vi "Connect.vi"(0 "Credentials":T1, 1 "Authenticate":bool=TRUE, 3 "error in (no error)":errorcluster) -> (6 "connection ID out":refnum<k5>, 7 "Connection Status":T4=enum."Connection refused: not authorized", 9 "error out":errorcluster)   [LabVIEW 2013, in "IOTFoundation.lvlib"]
uses:
  IOTFoundation.lvlib
  Controls/Connection_Return_Codes.ctl
  Controls/MessageType.ctl
  Controls/QoS.ctl
panel:
  out "QoS Level":T2
  out "MessageType":T3
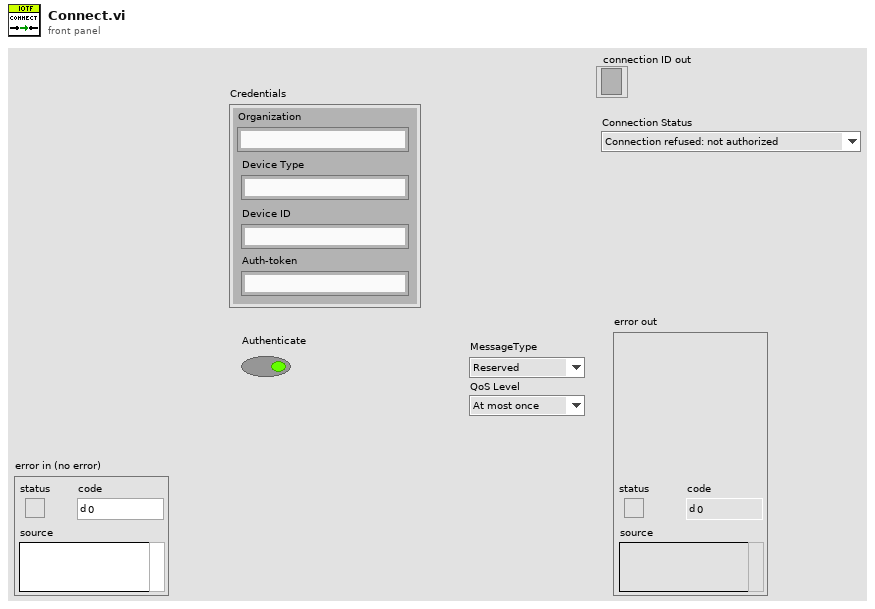
[diagram p1: front panel]
types:
  T1 = cluster{"Organization":string, "Device Type":string, "Device ID":string, "Auth-token":string}
  T2 = typedef "IOTFoundation.lvlib/QoS.ctl" = enum8{"At most once", "At least once", "Exactly once", "Reserved"}
  T3 = typedef "IOTFoundation.lvlib/MessageType.ctl" = enum32{"Reserved", "CONNECT", "CONNACK", "PUBLISH", "PUBACK", "PUBREC", "PUBREL", "PUBCOMP", "SUBSCRIBE", "SUBACK", "UNSUBSCRIBE", "UNSUBACK", "PINGREQ", "PINGRESP", "DISCONNECT", "Reserved2"}
  T4 = typedef "IOTFoundation.lvlib/Connection_Return_Codes.ctl" = enum16{"Connection accepted", "Connection refused: unacceptable protocol version", "Connection refused: identifier rejected", "Connection refused: Server unavailable", "Connection refused: bad user name or password", "Connection refused: not authorized"}
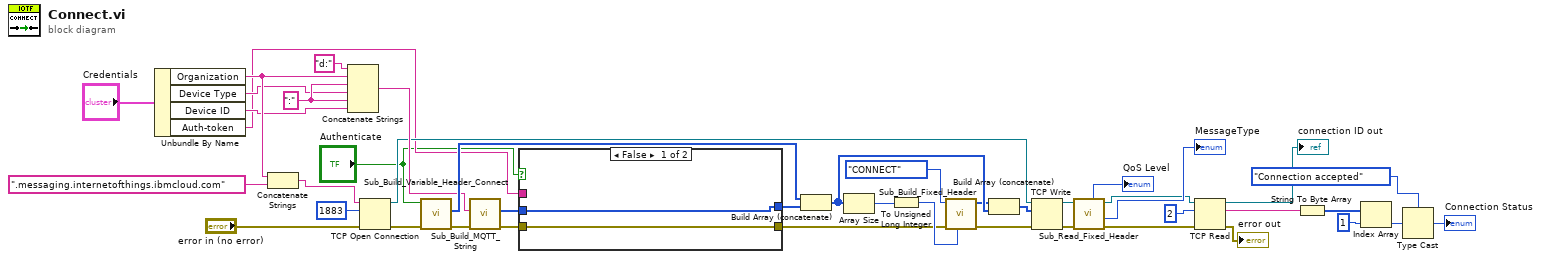
[diagram p0: block diagram]
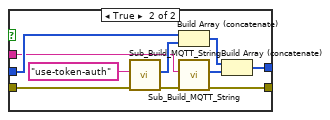
[diagram p2: hidden frame]
diagram:
  w30 = ":"
  n1 = Unbundle By Name("Credentials") -> ("Organization"=w5:string, "Device Type"=w4:string, "Device ID"=w3:string, "Auth-token"=w2:string)
  n2 = Concatenate Strings(w5, ".messaging.internetofthings.ibmcloud.com") -> (w26:string)
  n3 = Concatenate Strings("d:", w5, w30, w4, w30, w3) -> (w29:string)
  n4 = TCP Open Connection(address=w26, remote port or service name=1883, error in (no error)="error in (no error)") -> (connection ID=w23:refnum<k5>, error out=w27:errorcluster)  [unwired: 2 in]
  n5 = call "Sub_Build_Variable_Header_Connect.vi"("error in (no error)"=w27, "Authenticate"="Authenticate") -> ("error out"=w42:errorcluster, "Variable Header"=w41:u8[])  [unwired: 8 in]
  n6 = call "Sub_Build_MQTT_String.vi"("error in (no error)"=w42, "String to be encoded"=w29) -> ("error out"=w35:errorcluster, "UTF8 Byte Array"=w36:u8[])  [unwired: 8 in]
  n7 = case shown="False" "Authenticate" {
    tunnel: w36 -> [w44 w54]
    tunnel: w35 -> [w45 w53]
    tunnel: [w44 w49] -> w34
    tunnel: [w45 w48] -> w33
    tunnel: w2 -> [_ w47]
    frame False {
    }
    frame True {
      n8 = call "Sub_Build_MQTT_String.vi"("error in (no error)"=w53, "String to be encoded"="use-token-auth") -> ("error out"=w52:errorcluster, "UTF8 Byte Array"=w55:u8[])  [unwired: 8 in]
      n9 = Build Array (concatenate)(w54, w55) -> (w51:u8[])
      n10 = call "Sub_Build_MQTT_String.vi"("error in (no error)"=w52, "String to be encoded"=w47) -> ("error out"=w48:errorcluster, "UTF8 Byte Array"=w50:u8[])  [unwired: 8 in]
      n11 = Build Array (concatenate)(w51, w50) -> (w49:u8[])
    }
  }
  n12 = Build Array (concatenate)(w41, w34) -> (w40:u8[])
  n13 = Array Size(array=w40) -> (size(s)=w38:i32)
  n14 = To Unsigned Long Integer(number=w38) -> (unsigned 32bit integer=w37:u32)
  n15 = call "Sub_Build_Fixed_Header.vi"("Remaining Length"=w37, "error in (no error)"=w33, "MessageType"=MessageType."CONNECT") -> ("error out"=w24:errorcluster, "Fixed Header"=w39:u8[])  [unwired: 7 in]
  n16 = Build Array (concatenate)(w39, w40) -> (w22:u8[])
  n17 = TCP Write(connection ID=w23, data in=w22, error in (no error)=w24) -> (connection ID out=w11:refnum<k5>, error out=w10:errorcluster)  [unwired: 1 in, 1 out]
  n18 = call "Sub_Read_Fixed_Header.vi"("error in (no error)"=w10, "connection ID"=w11) -> ("error out"=w14:errorcluster, "MessageType"=→"MessageType":T3, "connection ID out"=w13:refnum<k5>, "QoS Level"=→"QoS Level":T2)  [unwired: 3 in, 3 out]
  n19 = TCP Read(connection ID=w13, bytes to read=2, error in (no error)=w14) -> (connection ID out=→"connection ID out":refnum<k5>, data out=w12:string, error out=→"error out":errorcluster)  [unwired: 2 in]
  n20 = String To Byte Array(string=w12) -> (unsigned byte array=w16:u8[])
  n21 = Index Array(array=w16, index=1) -> (element=w21:u8)
  n22 = Type Cast(type=Connection_Return_Codes."Connection accepted" ("Conn Return Code"), x=w21) -> (*(type *) &x=→"Connection Status":T4)
